vi "All-In-One_EIC-DIRC_DAQ.vi"() -> ()   [LabVIEW 2024]
uses:
  O:/DSG/Tyler/EIC/DIRC/daq/automated/Thorlabs.MotionControl.Controls.dll
  Thorlabs.MotionControl.Controls.dll
  <vilib>/numeric/Random Number (Range) DBL.vi
  O:/DSG/Tyler/EIC/DIRC/daq/automated/Thorlabs.MotionControl.IntegratedStepperMotorsCLI.dll
  Thorlabs.MotionControl.IntegratedStepperMotorsCLI.dll
  O:/DSG/Tyler/EIC/DIRC/daq/automated/Thorlabs.MotionControl.Benchtop.StepperMotorCLI.dll
  Thorlabs.MotionControl.Benchtop.StepperMotorCLI.dll
  <instrlib>/Keithley 6517/Keithley 6517.lvlib
panel:
  out "meter-mode":bool=TRUE
  in  "PDY start":dbl=105.8
  in  "PDX start":dbl=265.0
  out "run time (min)":dbl
  in  "align-only":bool
  out "alignment-counter":dbl=184.0 format="%#_13g"
  out "Optimized Location":dbl[](array[numeric])
  in  "N-M":bool
  in  "PD Y - in":cluster{"start":dbl, "stop":dbl, "step":dbl}={"start"=126.5, "stop"=128.5, "step"=2.0}
  in  "PD X - in":cluster{"start":dbl, "stop":dbl, "step":dbl}={"start"=268.0, "stop"=270.0, "step"=2.0}
  in  "out-pda":dbl=180.5 caption="Bar Out - PD Angle" format="%#_13g"
  in  "out-bma":dbl=45.0 caption="Bar Out - Brewster Angle" format="%#_13g"
  in  "out-bar-y":dbl=20.0 caption="Bar Out - Bar Y pos." format="%#_13g"
  in  "out-bar-x":dbl=93.0 caption="Bar Out - Bar X pos." format="%#_13g"
  in  "scan-v2":bool
  in  "in-pda":dbl=180.5 caption="Bar In - PD Angle" format="%#_13g"
  in  "in-bma":dbl=45.0 caption="Bar In - Brewster Angle" format="%#_13g"
  in  "Test Start Delay (s)":dbl=30.0
  in  "Bar Y - in":cluster{"start":dbl, "stop":dbl, "step":dbl}={"start"=20.0, "stop"=22.0, "step"=2.0}
  in  "Bar X - in":cluster{"start":dbl, "stop":dbl, "step":dbl}={"start"=235.0, "stop"=237.0, "step"=2.0}
  in  "PD Y - out":cluster{"start":dbl, "stop":dbl, "step":dbl}={"start"=126.5, "stop"=128.5, "step"=2.0}
  in  "PD X - out":cluster{"start":dbl, "stop":dbl, "step":dbl}={"start"=268.0, "stop"=270.0, "step"=2.0}
  out "Queue % Left":dbl format="%#_3g"
  out "next-state-cluster-const":T1={"next-state"="", "bypass-confirm"=FALSE, "PDX"=300.0, "PDY"=150.0, "BarX"=300.0, "BarY"=150.0, "BMA"=45.0, "PDA"=85.0, "bar-note"=FALSE}
  in  "X start":dbl=262.0
  in  "X end":dbl=263.0
  in  "Y end":dbl=121.5 format="%#_13g"
  in  "X step size":dbl=0.2 format="%#_13g"
  in  "Y step size":dbl=0.2
  in  "Y start":dbl=120.5 format="%#_13g"
  in  "diode-scan":bool
  out "keep-file":bool
  out "status":string
  out "queue-size":i32
  in  "save-loc":bool
  out "stored-pos":T2 caption="Location Stored"
  out "main-stage-refs":T3
  out "state-queue":T4(array[cluster])
  in  "PDA":dbl=184.0 format="%#_13g"
  in  "BMA":dbl=45.0 format="%#_13g"
  in  "BarY":dbl=30.0 format="%#_13g"
  in  "BarX":dbl=230.0 format="%#_13g"
  in  "PDY":dbl=124.0 format="%#_13g"
  in  "PDX":dbl=274.0 format="%#_13g"
  out "bypass-confirm":bool
  out "PD Values":cluster{"PD1":dbl, "PD2":dbl, "PD3":dbl}
  out "last-PD":dbl[](array[numeric])=[1.0, 1.0, 1.0]
  in  "move-bar":bool
  in  "multi-trial":bool
  out "pd_angle":dbl
  out "brewster_angle":dbl
  out "meter-visa":refnum<visa-resource-name>
  out "loop-rate":u32
  out "meter-stat":bool caption="Log Status"
  out "file-stat":bool caption="Log Status"
  out "stage-stat":bool caption="Log Status"
  out "last-save-time":string caption="Time of Last Save:"
  out "pd_y_pos":dbl
  out "pd_x_pos":dbl
  out "bar_y_pos":dbl
  out "bar_x_pos":dbl
  in  "nSamples":dbl=50.0 caption="# Samples"
  out "Current Time:":string
  in  "save-data":bool
  in  "bar-note":bool
  out "pd3_v":dbl caption="PD 3" format="%#.4g"
  out "pd2_v":dbl caption="PD 2" format="%#.4g"
  out "pd1_v":dbl caption="PD 1" format="%#.4g"
  out "meter-error":errorcluster
  out "log-error":errorcluster
  out "log-path":path caption="Path Data Will Save To:"
  out "start-msg":string
  out "stage-error":errorcluster
  in  "PD Angle":refnum<k24>(container)
  in  "Brewster":refnum<k24>(container)
  in  "PD Y":refnum<k24>(container)
  in  "PD X":refnum<k24>(container)
  in  "BAR Y":refnum<k24>(container)
  in  "stop":bool
  in  "BAR X":refnum<k24>(container)
  out "pd-plt":cluster{"[0]":dbl, "[1]":dbl, "[2]":dbl}(graph) caption="Measurement History"
  # "EXPERT DEBUGGING INFO"
  # "A"
  # "A"
  # "A"
  # "Work In Progress - please do not use"
  # "PD + BAR SCAN"
  # "BAR OUT SETTINGS"
  # "BAR IN SETTINGS"
  # "PD ONLY SCAN - CENTERED"
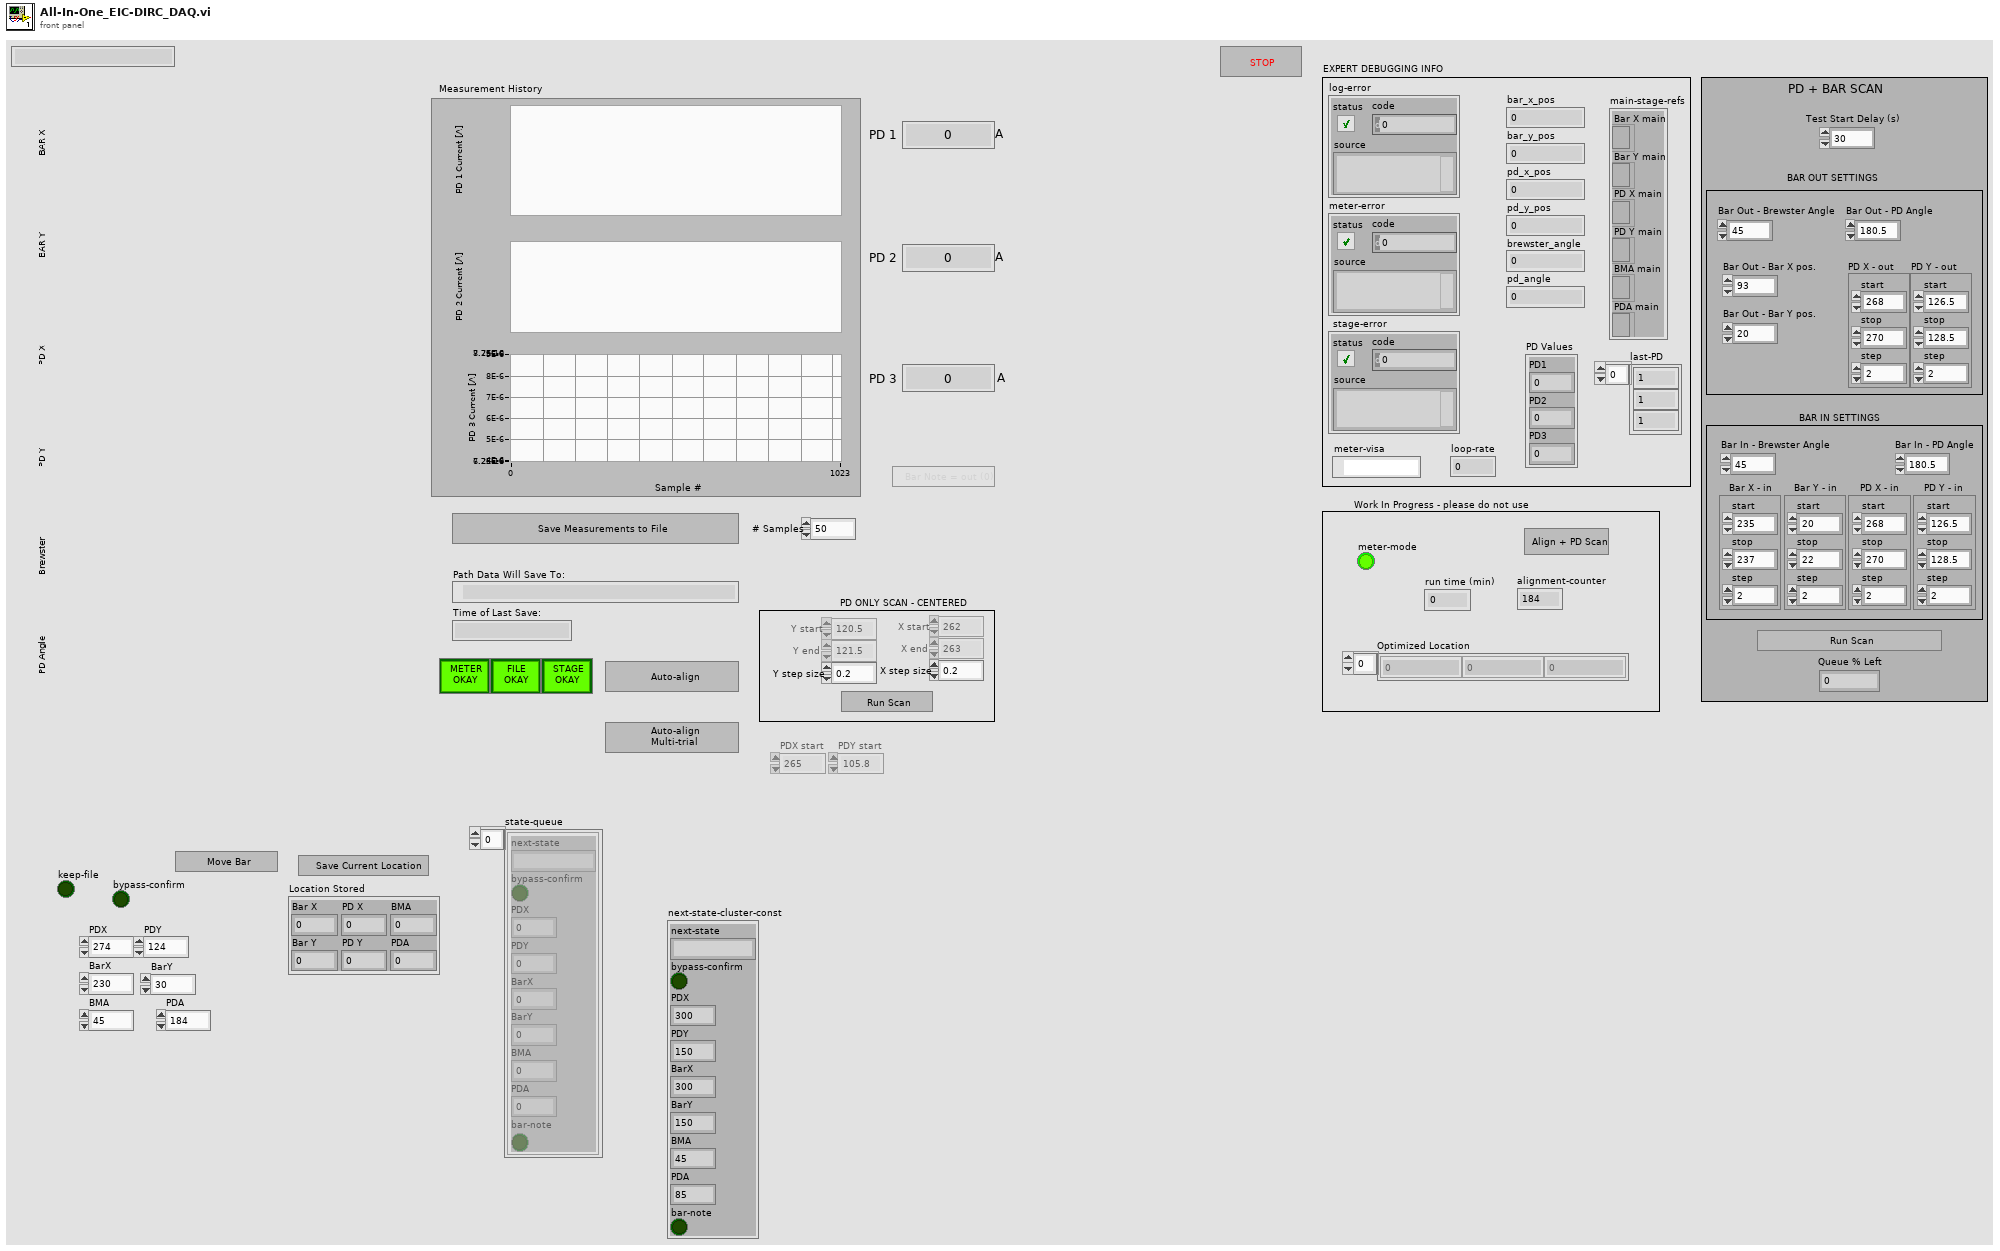
[diagram p1: front panel]
types:
  T1 = cluster{"next-state":string, "bypass-confirm":bool, "PDX":dbl, "PDY":dbl, "BarX":dbl, "BarY":dbl, "BMA":dbl, "PDA":dbl, "bar-note":bool}
  T2 = cluster{"Bar X":dbl, "Bar Y":dbl, "PD X":dbl, "PD Y":dbl, "BMA":dbl, "PDA":dbl}
  T3 = cluster{"Bar X main":refnum<k24>, "Bar Y main":refnum<k24>, "PD X main":refnum<k24>, "PD Y main":refnum<k24>, "BMA main":refnum<k24>, "PDA main":refnum<k24>}
  T4 = cluster{"next-state":string, "bypass-confirm":bool, "PDX":dbl, "PDY":dbl, "BarX":dbl, "BarY":dbl, "BMA":dbl, "PDA":dbl, "bar-note":bool}[]
  T5 = cluster{"Bar X":refnum<k24>, "Bar Y":refnum<k24>, "PD X":refnum<k24>, "PD Y":refnum<k24>, "Brewster":refnum<k24>, "PD Angle":refnum<k24>}
  T6 = enum16{"open", "replace", "create", "open or create", "replace or create", "replace or create with confirmation"}
  T7 = cluster{"alpha":dbl, "gamma":dbl, "rho":dbl, "sigma":dbl, "simplex L":dbl}
  T8 = cluster{"next-state":string, "mode-select":enum32{"IR", "Pure", "Bulk", "Bar Out", "stored-loc", "custom"}, "bypass-confirm":bool, "PDX":dbl, "PDY":dbl, "BarX":dbl, "BarY":dbl, "BMA":dbl, "PDA":dbl, "bar-note":bool}
  T9 = cluster{"error":bool, "code":i32, "source":string}
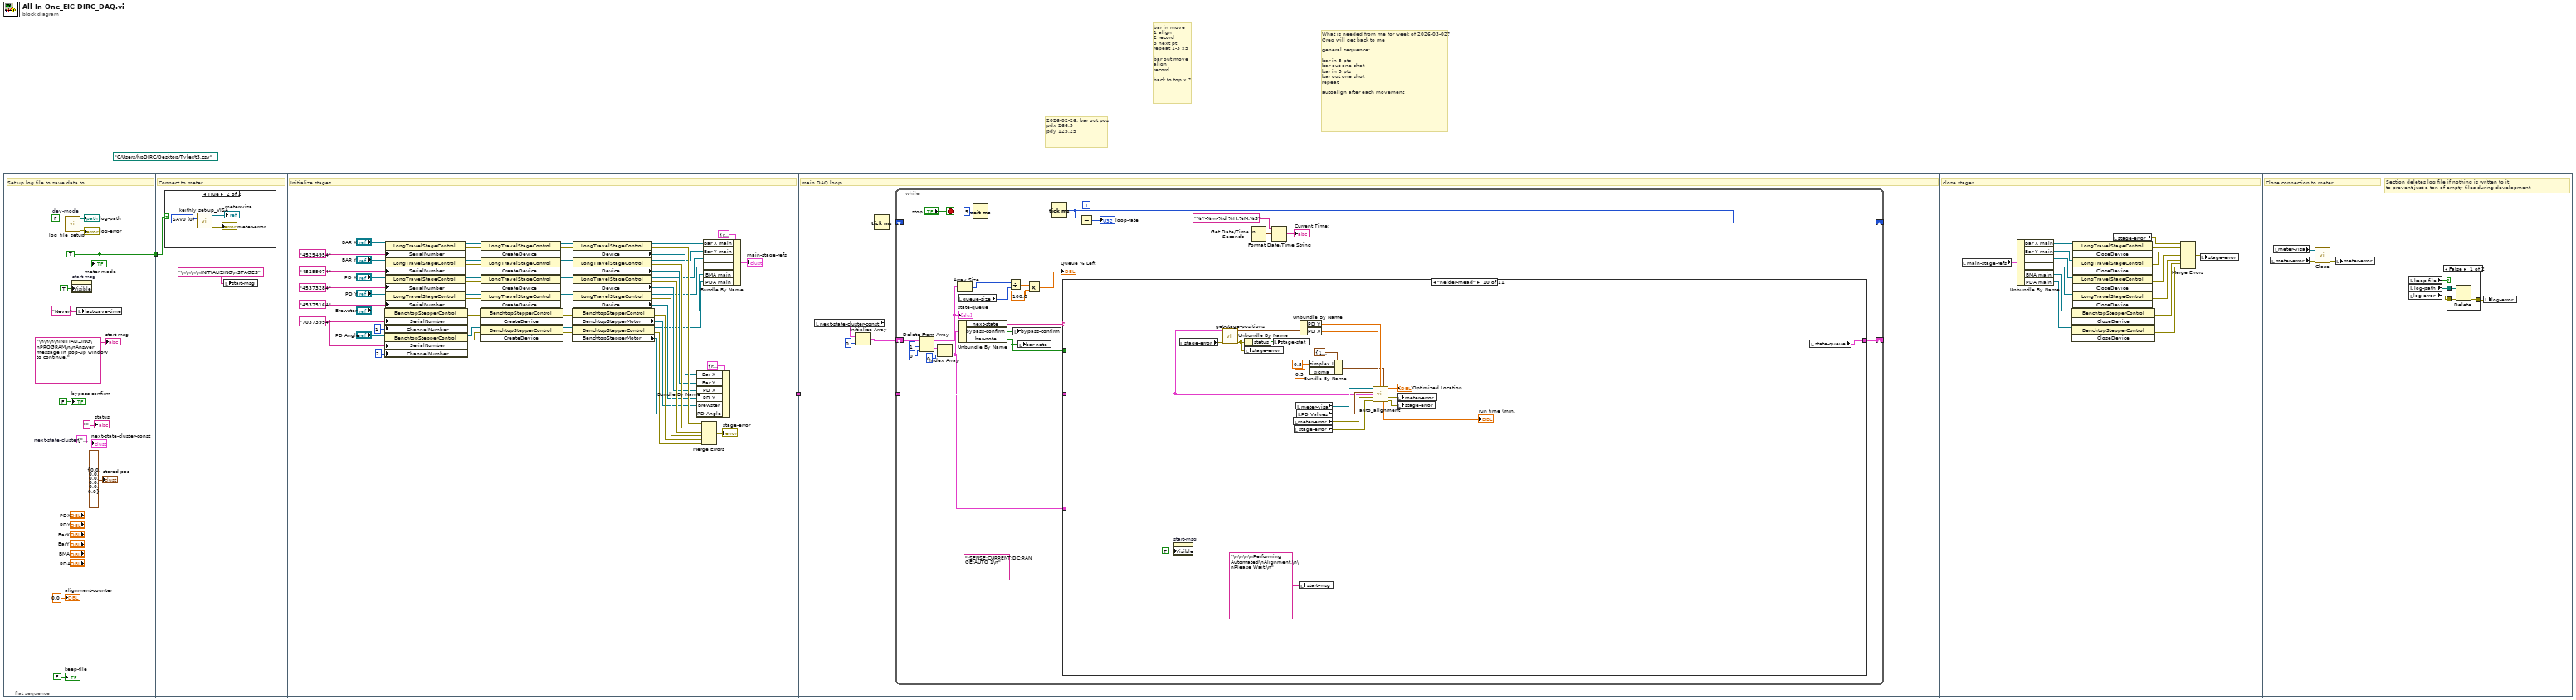
[diagram p0: block diagram]
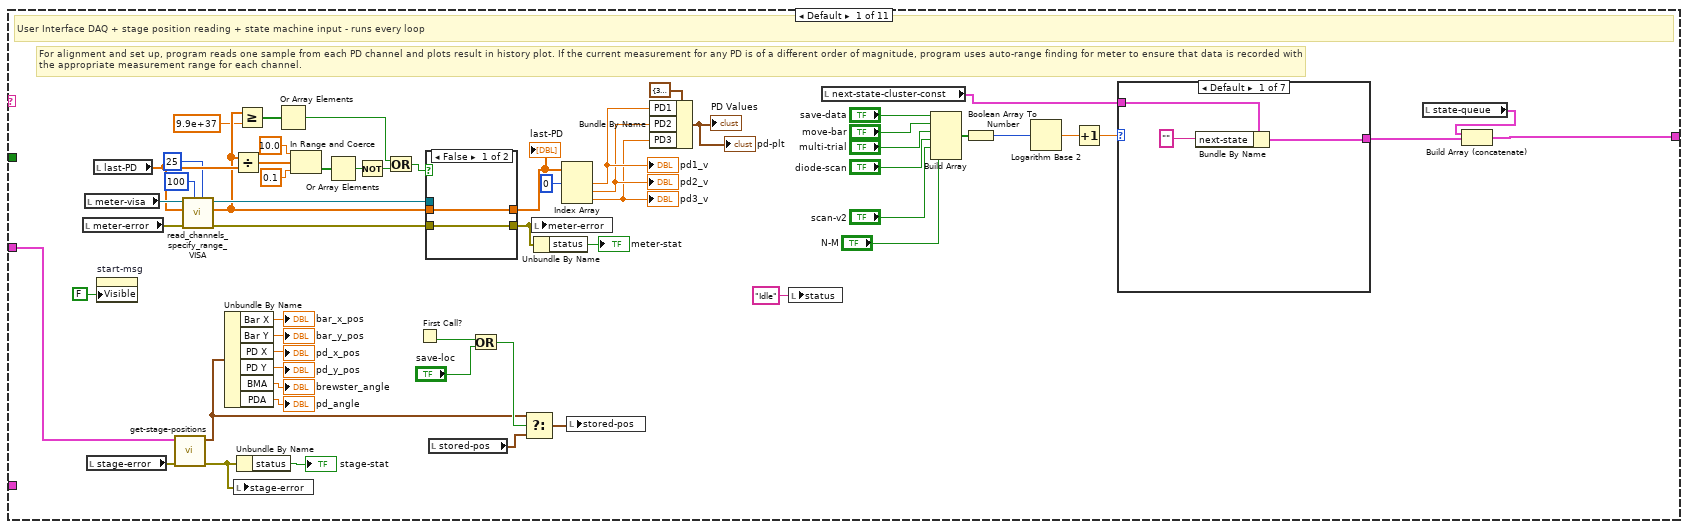
[diagram p3: hidden frame]
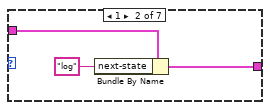
[diagram p4: hidden frame]
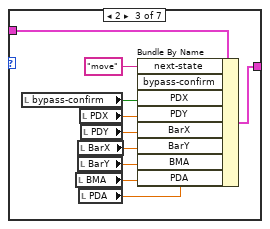
[diagram p5: hidden frame]
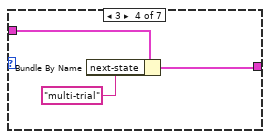
[diagram p6: hidden frame]
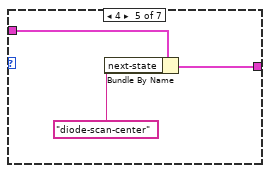
[diagram p7: hidden frame]
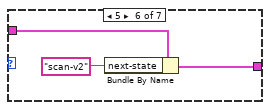
[diagram p8: hidden frame]
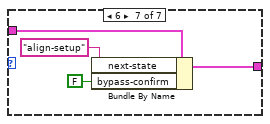
[diagram p9: hidden frame]
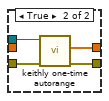
[diagram p10: hidden frame]
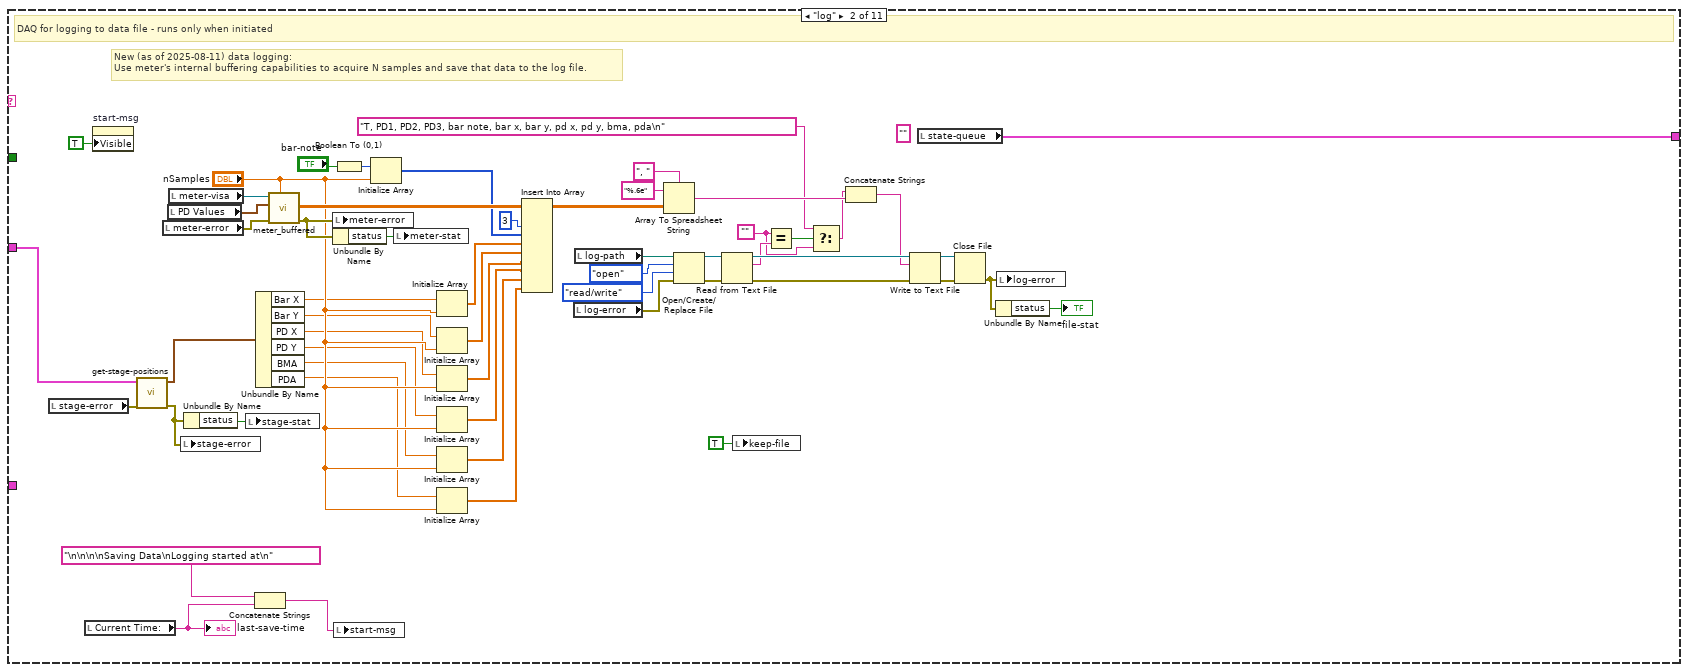
[diagram p11: hidden frame]
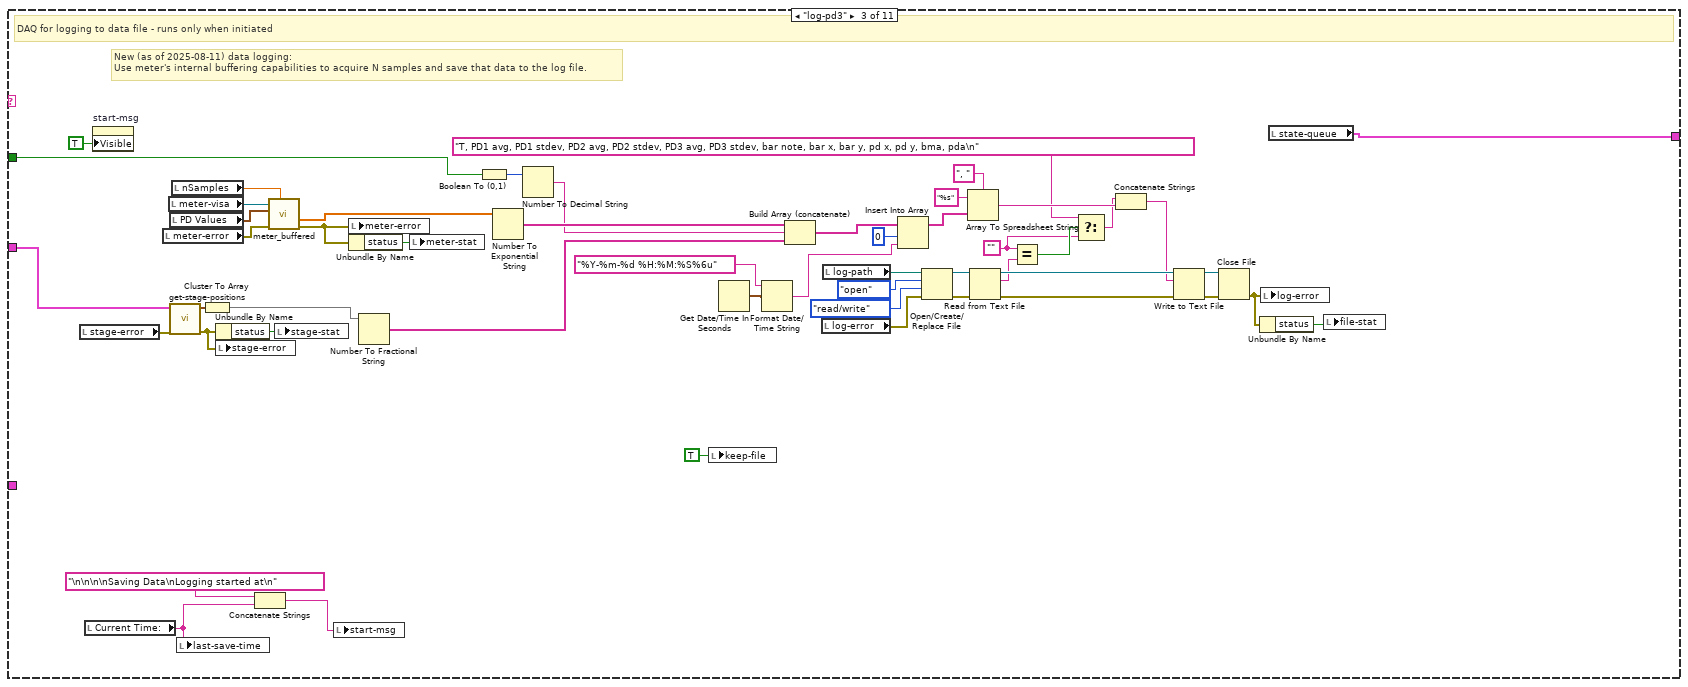
[diagram p12: hidden frame]
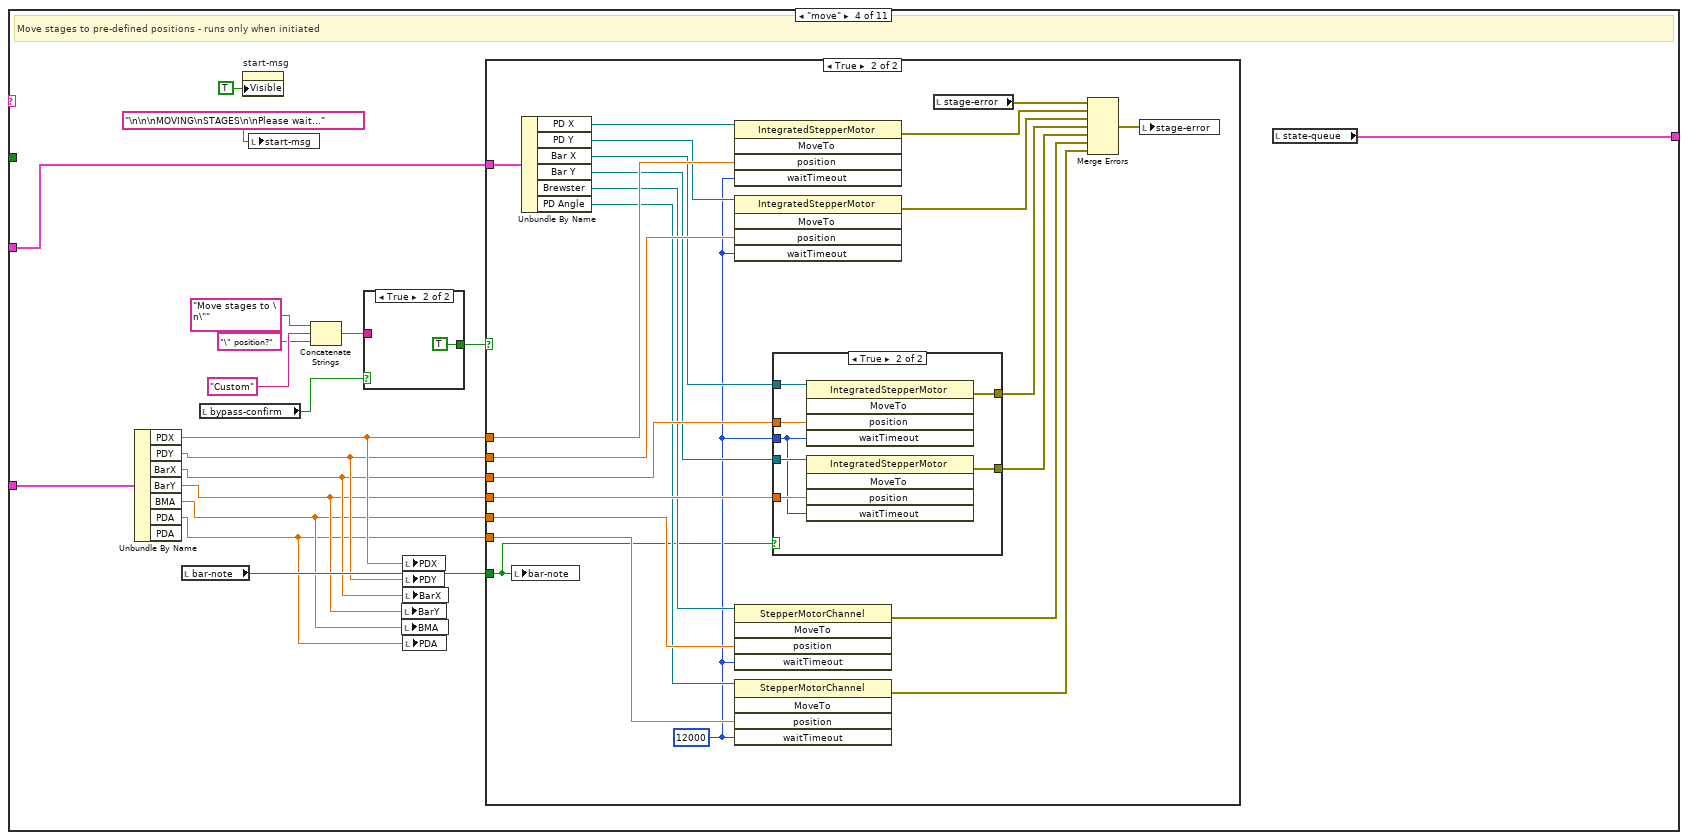
[diagram p13: hidden frame]
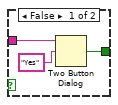
[diagram p14: hidden frame]
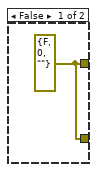
[diagram p16: hidden frame]
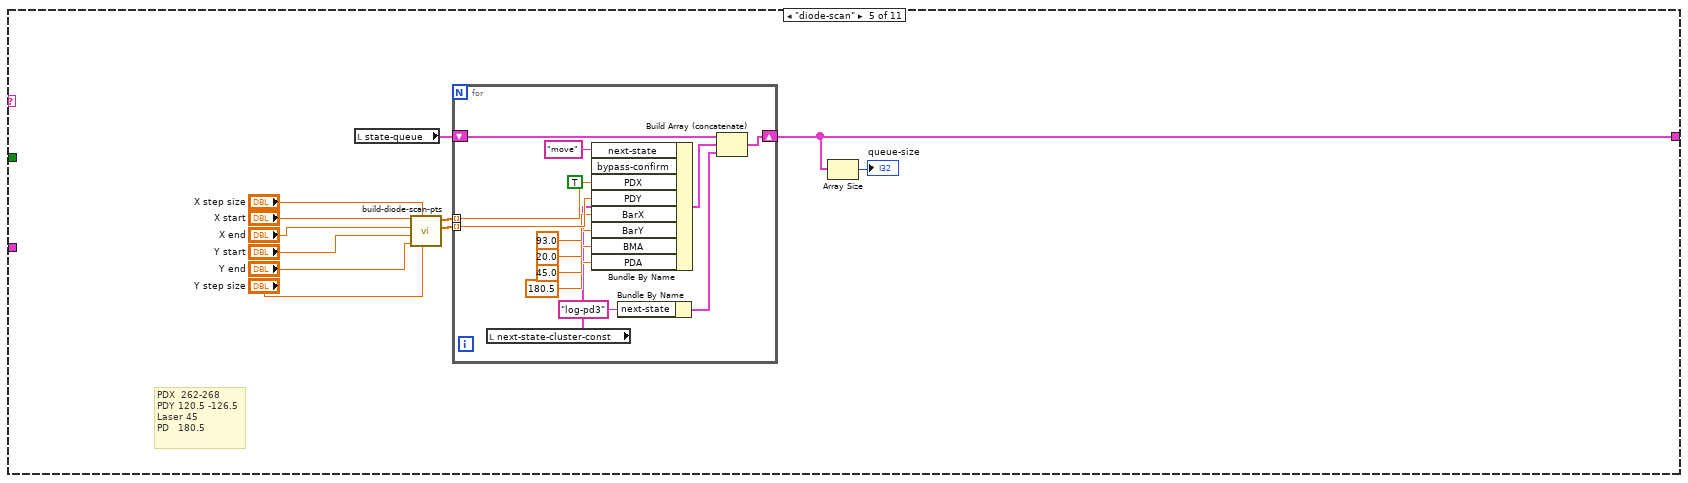
[diagram p17: hidden frame]
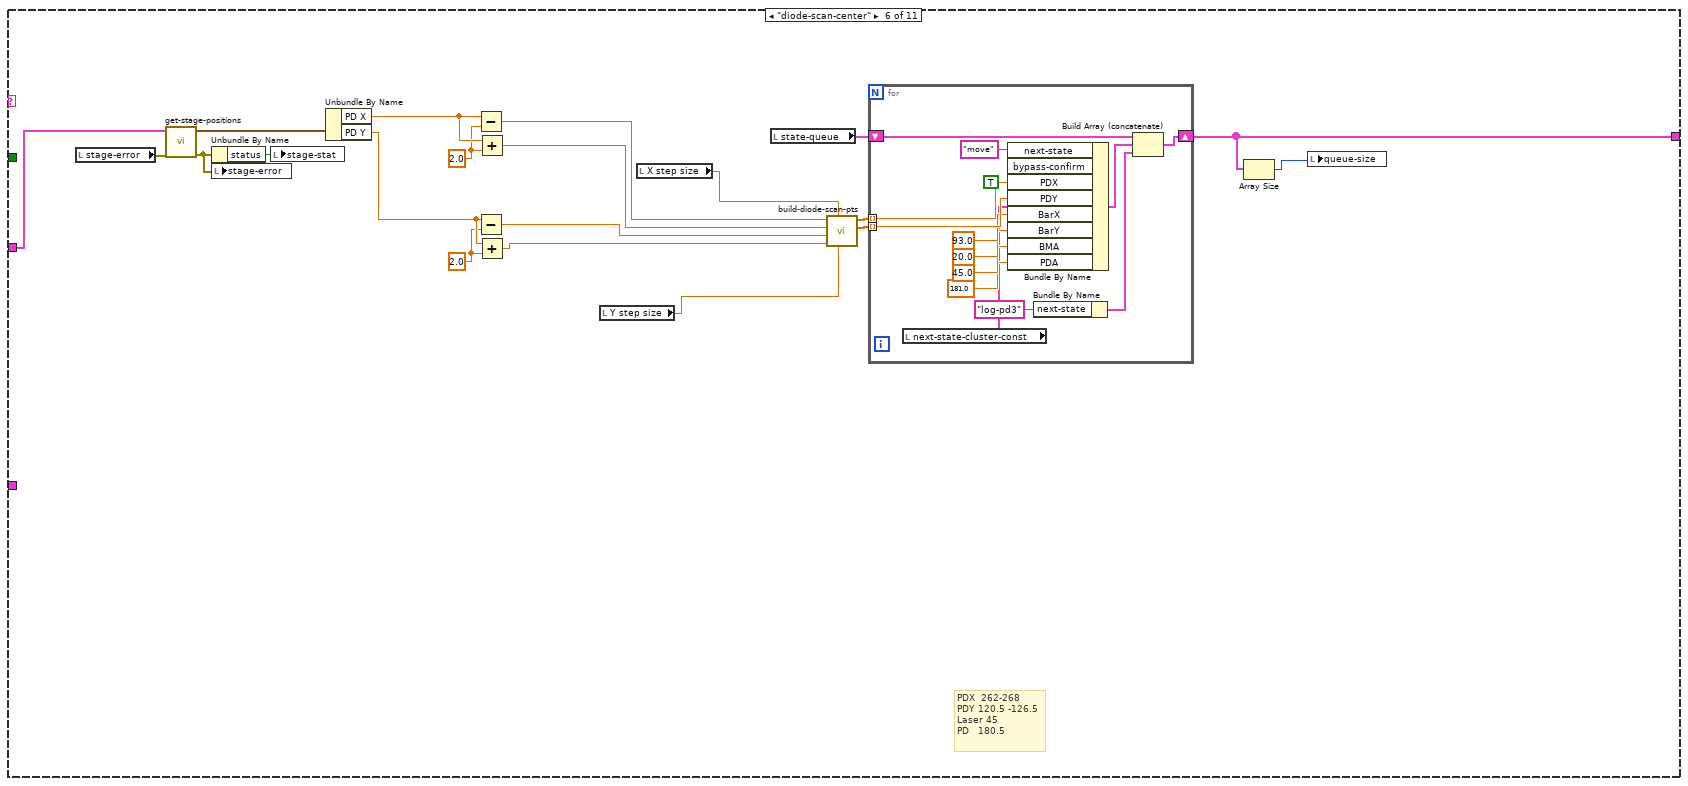
[diagram p18: hidden frame]
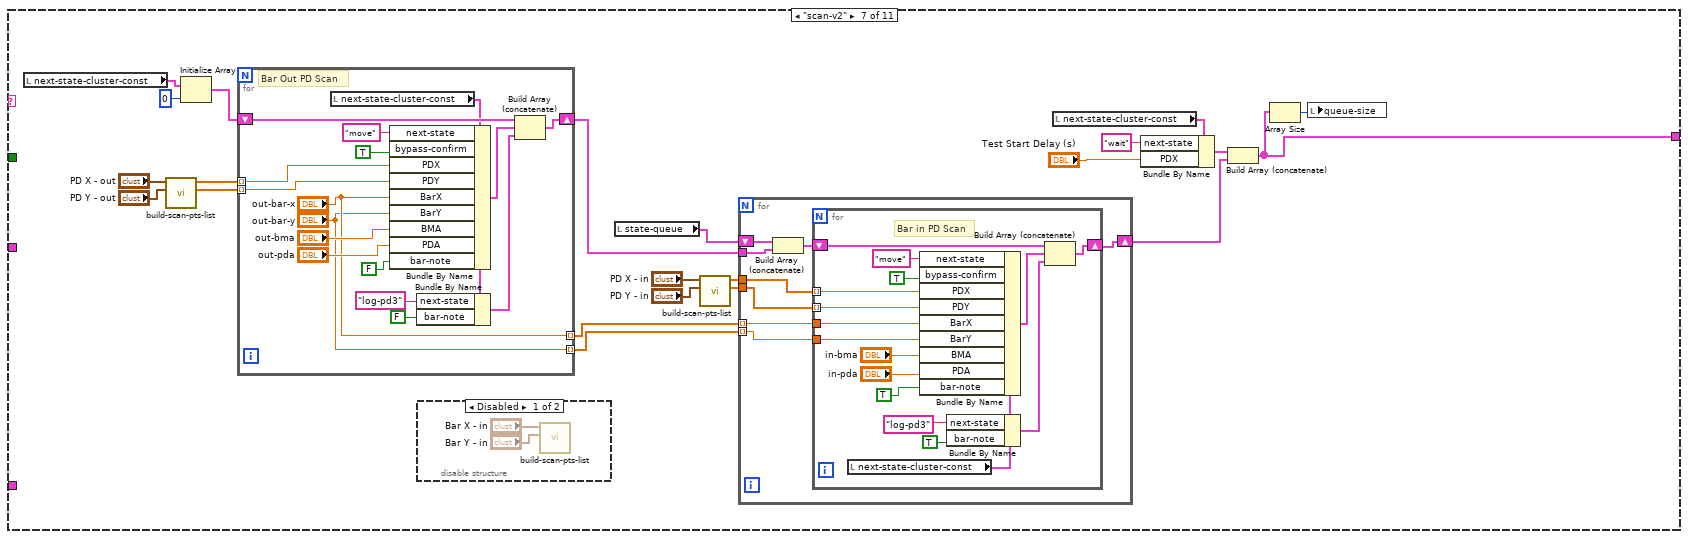
[diagram p19: hidden frame]
diagram:
  (unwired) path "C:/Users/hpDIRC/Desktop/Tyler/t3.csv" ("log-path")
  # "2026-02-26: bar out pos\npdx 266.5\npdy 125.25"
  # "bar in move\n1 align\n2 record\n3 next pt\nrepeat 1-3 x5\n\nbar out move\nalign\nrecord\n\nback to top x ?"
  # "What is needed from me for week of 2026-03-02?\nGreg will get back to me\n\ngeneral sequence:\n\nbar in 5 pts \nbar out one shot\nbar in 5 pts\nbar out one shot\nrepeat\n\nautoalign after each movement"
  n1 = flat-sequence {
    tunnel: [w3] -> w1
    tunnel: w1 -> [w15]
    tunnel: [w28] -> w2
    tunnel: w2 -> [w80]
    frame #0 {
      w3 = TRUE
      (unwired) T8 {"next-state"="", "mode-select"=enum."IR", "bypass-confirm"=FALSE, "PDX"=300.0, "PDY"=150.0, "BarX"=300.0, "BarY"=150.0, "BMA"=45.0, "PDA"=85.0, "bar-note"=FALSE}  # next-state-cluster
      w14 = FALSE  # dev-mode
      # "Set up log file to save data to"
      n2 = call "log_file_setup.vi"("dev-mode"=w14) -> ("error out"=→"log-error":errorcluster, "appended path"=→"log-path":path)  [unwired: 8 in, 1 out]
      n3 = property on="start-msg" class="Str"("Visible"=TRUE) -> ()  [unwired: 2 in, 2 out]
      n4 = local write "last-save-time"("Never" ("date/time string")) -> ()
      "start-msg" <- "\n\n\n\nINITIALIZING\nPROGRAM\n\nAnswer message in pop-up window to continue." ("String")
      "bypass-confirm" <- FALSE
      "stored-pos" <- T2 {"Bar X"=0.0, "Bar Y"=0.0, "PD X"=0.0, "PD Y"=0.0, "BMA"=0.0, "PDA"=0.0} ("stage-pos")
      "status" <- "" ("status")
      "keep-file" <- FALSE
      "alignment-counter" <- 0.0 ("alignment-counter")
      "meter-mode" <- w3
    }
    frame #1 {
      # "Connect to meter"
      n5 = case shown="True" w15 {
        frame False {
        }
        frame True {
          w17 = i16 0 items=["SAV0", "SAV1", "SAV2", "SAV3", "SAV4", "SAV5", "SAV6", "SAV7", "SAV8", "SAV9", "RST", "Preset"] ("ConfigOpt")
          n6 = call "keithly set-up_VISA.vi"("ConfigOpt"=w17) -> ("error out"=→"meter-error":errorcluster, "meter-VISA"=→"meter-visa":refnum<visa-resource-name>)  [unwired: 9 in]
        }
      }
      n7 = local write "start-msg"("\n\n\n\nINITIALIZING\nSTAGES" ("String")) -> ()
    }
    frame #2 {
      w35 = "70373994" ("SerialNumber")
      # "Initialize stages"
      n8 = property class="BenchtopStepperControl"(reference="Brewster", "SerialNumber"=w35, "ChannelNumber"=1) -> (reference out=w61:refnum<k24>, error out=w62:errorcluster)  [unwired: 1 in]
      n9 = property class="BenchtopStepperControl"(reference="PD Angle", "SerialNumber"=w35, "ChannelNumber"=2) -> (reference out=w60:refnum<k24>, error out=w63:errorcluster)  [unwired: 1 in]
      n10 = property class="LongTravelStageControl"(reference="BAR X", "SerialNumber"="45294954") -> (reference out=w38:refnum<k24>, error out=w45:errorcluster)  [unwired: 1 in]
      n11 = property class="LongTravelStageControl"(reference="BAR Y", "SerialNumber"="45299074") -> (reference out=w39:refnum<k24>, error out=w46:errorcluster)  [unwired: 1 in]
      n12 = property class="LongTravelStageControl"(reference="PD X", "SerialNumber"="45373284") -> (reference out=w42:refnum<k24>, error out=w47:errorcluster)  [unwired: 1 in]
      n13 = property class="LongTravelStageControl"(reference="PD Y", "SerialNumber"="45375164") -> (reference out=w43:refnum<k24>, error out=w48:errorcluster)  [unwired: 1 in]
      n14 = invoke class="BenchtopStepperControl" method="CreateDevice"(reference=w61, error in=w62) -> (reference out=w58:refnum<k24>, error out=w56:errorcluster)  [unwired: 1 in, 1 out]
      n15 = invoke class="BenchtopStepperControl" method="CreateDevice"(reference=w60, error in=w63) -> (reference out=w57:refnum<k24>, error out=w59:errorcluster)  [unwired: 1 in, 1 out]
      n16 = invoke class="LongTravelStageControl" method="CreateDevice"(reference=w38, error in=w45) -> (reference out=w51:refnum<k24>, error out=w55:errorcluster)  [unwired: 1 in, 1 out]
      n17 = invoke class="LongTravelStageControl" method="CreateDevice"(reference=w39, error in=w46) -> (reference out=w52:refnum<k24>)  [unwired: 1 in, 2 out]
      n18 = invoke class="LongTravelStageControl" method="CreateDevice"(reference=w42, error in=w47) -> (reference out=w53:refnum<k24>)  [unwired: 1 in, 2 out]
      n19 = invoke class="LongTravelStageControl" method="CreateDevice"(reference=w43, error in=w48) -> (reference out=w54:refnum<k24>)  [unwired: 1 in, 2 out]
      n20 = property class="BenchtopStepperControl"(reference=w58, error in=w56) -> (reference out=w22:refnum<k24>, error out=w73:errorcluster, "BenchtopStepperMotor"=w68:refnum<k24>)
      n21 = property class="BenchtopStepperControl"(reference=w57, error in=w59) -> (reference out=w21:refnum<k24>, error out=w74:errorcluster, "BenchtopStepperMotor"=w69:refnum<k24>)
      n22 = property class="LongTravelStageControl"(reference=w51, error in=w55) -> (reference out=w26:refnum<k24>, error out=w75:errorcluster, "Device"=w64:refnum<k24>)
      n23 = property class="LongTravelStageControl"(reference=w52) -> (reference out=w25:refnum<k24>, error out=w70:errorcluster, "Device"=w65:refnum<k24>)  [unwired: 1 in]
      n24 = property class="LongTravelStageControl"(reference=w53) -> (reference out=w24:refnum<k24>, error out=w71:errorcluster, "Device"=w66:refnum<k24>)  [unwired: 1 in]
      n25 = property class="LongTravelStageControl"(reference=w54) -> (reference out=w23:refnum<k24>, error out=w72:errorcluster, "Device"=w67:refnum<k24>)  [unwired: 1 in]
      n26 = Bundle By Name(cluster=T5 {"Bar X"=refnum, "Bar Y"=refnum, "PD X"=refnum, "PD Y"=refnum, "Brewster"=refnum, "PD Angle"=refnum}, "Bar X"=w64, "Bar Y"=w65, "PD X"=w66, "PD Y"=w67, "Brewster"=w68, "PD Angle"=w69) -> (w28:T5)
      n27 = Merge Errors(w75, w70, w71, w72, w73, w74) -> (→"stage-error":errorcluster)
      n28 = Bundle By Name(cluster=T3 {"Bar X main"=refnum, "Bar Y main"=refnum, "PD X main"=refnum, "PD Y main"=refnum, "BMA main"=refnum, "PDA main"=refnum}, "Bar X main"=w26, "Bar Y main"=w25, "PD X main"=w24, "PD Y main"=w23, "BMA main"=w22, "PDA main"=w21) -> (→"main-stage-refs":T3)
    }
    frame #3 {
      # "main DAQ loop"
      n29 = local read "next-state-cluster-const"() -> (w77:T1)
      n30 = Initialize Array(w77, 0 ("dimension size")) -> (w79:T4)
      n31 = Tick Count (ms)() -> (millisecond timer value=w81:u32)
      n32 = while {
        shift-right: [w105] -> _
        shift-left: w81 -> [w104]
        tunnel: w80 -> [w102]
        shift-right: [w90] -> _
        shift-left: w79 -> [w92]
        stop <- "stop" stop-if-true
        (unwired) ":SENSE:CURRENT:DC:RANGE:AUTO 1\n"
        n33 = Delete From Array(array=w92, length=1, index=0) -> (deleted portion=w91:T4, array with subset deleted=w88:T4)
        "state-queue" <- w88
        n34 = Index Array(array=w91, index=0) -> (element=w89:T1)
        n35 = Array Size(array=w88) -> (size(s)=w83:i32)
        n36 = local read "queue-size"() -> (w87:i32)
        n37 = Unbundle By Name(w89) -> ("next-state"=w94:string, "bypass-confirm"=w93:bool, "bar-note"=w82:bool)
        n38 = Wait (ms)(milliseconds to wait=u32 5) -> ()  [unwired: 1 out]
        n39 = Divide(x=w83, y=w87) -> (x/y=w86:dbl)
        n40 = local write "bypass-confirm"(w93) -> ()
        n41 = local write "bar-note"(w82) -> ()
        n42 = Multiply(x=w86, y=100.0) -> (x*y=→"Queue % Left":dbl)
        n43 = Tick Count (ms)() -> (millisecond timer value=w105:u32)
        n44 = case shown="\"nelder-mead\"" w94 {
          tunnel: w102 -> [w157 w218 w286 w319 _ w394 _ _ _ w526 _]
          tunnel: [w128 w229 w291 w317 w368 w402 w428 w486 w492 w534 w537] -> w90
          tunnel: w89 -> [_ _ _ w314 _ _ _ w487 w497 _ _]
          tunnel: w82 -> [_ _ w269 _ _ _ _ _ _ _ _]
          frame Default {
            # "For alignment and set up, program reads one sample from each PD channel and plots result in history plot. If the current measurement for any PD is of a different order of magnitude, program uses auto-range finding for meter to ensure that data is recorded with the appropriate measurement range for each channel."
            # "User Interface DAQ + stage position reading + state machine input - runs every loop"
            n45 = local read "meter-error"() -> (w154:errorcluster)
            n46 = local read "meter-visa"() -> (w155:refnum<visa-resource-name>)
            n47 = local read "stage-error"() -> (w156:errorcluster)
            n48 = local read "last-PD"() -> (w145:dbl[])
            n49 = property on="start-msg" class="Str"("Visible"=FALSE) -> ()  [unwired: 2 in, 2 out]
            n50 = call "get-stage-positions.vi"("error in (no error)"=w156, "Cluster"=w157) -> ("error out"=w142:errorcluster, "stage positions"=w114:T2)  [unwired: 8 in]
            n51 = call "read_channels_specify_range_VISA.vi"("postDAQ  wait ms"=u32 25, "preDAQ  wait ms"=u32 100, "error in"=w154, "range"=w145, "VISA resource in"=w155) -> ("error out"=w147:T9, "data"=w134:dbl[], "VISA resource out"=w146:refnum<visa-resource-name>)  [unwired: 4 in]
            n52 = Unbundle By Name(w114) -> ("Bar X"=→"bar_x_pos":dbl, "Bar Y"=→"bar_y_pos":dbl, "PD X"=→"pd_x_pos":dbl, "PD Y"=→"pd_y_pos":dbl, "BMA"=→"brewster_angle":dbl, "PDA"=→"pd_angle":dbl)
            n53 = Divide(x=w134, y=w145) -> (x/y=w150:dbl[])
            n54 = local write "stage-error"(w142) -> ()
            n55 = Greater Or Equal?(x=w134, y=9.9e+37) -> (x >= y?=w132:bool[])
            n56 = Unbundle By Name(w142) -> ("status"=→"stage-stat":bool)
            n57 = Or Array Elements(Boolean array=w132) -> (logical OR=w131:bool)
            n58 = In Range and Coerce(upper limit=10.0, x=w150, lower limit=0.1) -> (In Range?=w148:bool[])  [unwired: 1 out]
            n59 = Or Array Elements(Boolean array=w148) -> (logical OR=w149:bool)
            n60 = Not(x=w149) -> (.not. x?=w136:bool)
            n61 = Or(x=w131, y=w136) -> (x .or. y?=w135:bool)
            n62 = First Call?() -> (First Call?: T/F=w124:bool)
            n63 = case shown="False" w135 {
              tunnel: w147 -> [w196 w200]
              tunnel: [w196 w199] -> w163
              tunnel: [w195 w198] -> w158
              tunnel: w134 -> [w195 _]
              tunnel: w146 -> [_ w197]
              frame False {
              }
              frame True {
                n64 = call "keithly one-time autorange.vi"("error in"=w200, "VISA in"=w197) -> ("error out"=w199:errorcluster, "data"=w198:dbl[])  [unwired: 7 in, 1 out]
              }
            }
            "last-PD" <- w158
            n65 = local read "stored-pos"() -> (w125:T2)
            n66 = Or(x=w124, y="save-loc") -> (x .or. y?=w122:bool)
            n67 = Select(t=w114, s=w122, f=w125) -> (s? t:f=w126:T2)
            n68 = local write "meter-error"(w163) -> ()
            n69 = Unbundle By Name(w163) -> ("status"=→"meter-stat":bool)
            n70 = Index Array(array=w158, index #1=0 ("index")) -> (element #1=w161:dbl, element #2=w160:dbl, element #3=w159:dbl)  [unwired: 2 in]
            "pd3_v" <- w159
            "pd2_v" <- w160
            "pd1_v" <- w161
            n71 = local write "stored-pos"(w126) -> ()
            n72 = Bundle By Name(cluster=cluster{"PD1":dbl, "PD2":dbl, "PD3":dbl} {"PD1"=3e-05, "PD2"=3e-05, "PD3"=3e-05} ("PD ranges"), "PD1"=w161, "PD2"=w160, "PD3"=w159) -> (→"pd-plt" →"PD Values":cluster{"PD1":dbl, "PD2":dbl, "PD3":dbl})
            n73 = local write "status"("Idle" ("status")) -> ()
            n74 = local read "next-state-cluster-const"() -> (w112:T1)
            n75 = Build Array("save-data", "move-bar", "multi-trial", "diode-scan", "scan-v2", "N-M") -> (w138:bool[])
            n76 = Boolean Array To Number(Boolean array=w138) -> (number=w108:u32)
            n77 = Logarithm Base 2(1:w108) -> (0:w110:dbl)
            n78 = Increment(x=w110) -> (x+1=w109:dbl)
            n79 = case shown="Default" w109 {
              tunnel: w112 -> [w168 w171 w181 w184 w187 w190 w193]
              tunnel: [w166 w169 w179 w182 w185 w188 w194] -> w127
              frame Default {
                n80 = Bundle By Name(cluster=w168, "next-state"="") -> (w166:T1)
              }
              frame 1 {
                n81 = Bundle By Name(cluster=w171, "next-state"="log") -> (w169:T1)
              }
              frame 2 {
                n82 = local read "bypass-confirm"() -> (w172:bool)
                n83 = local read "BMA"() -> (w177:dbl)
                n84 = local read "BarX"() -> (w175:dbl)
                n85 = local read "BarY"() -> (w176:dbl)
                n86 = local read "PDA"() -> (w178:dbl)
                n87 = local read "PDX"() -> (w173:dbl)
                n88 = local read "PDY"() -> (w174:dbl)
                n89 = Bundle By Name(cluster=w181, "next-state"="move", "bypass-confirm"=w172, "PDX"=w173, "PDY"=w174, "BarX"=w175, "BarY"=w176, "BMA"=w177, "PDA"=w178) -> (w179:T1)
              }
              frame 3 {
                n90 = Bundle By Name(cluster=w184, "next-state"="multi-trial") -> (w182:T1)
              }
              frame 4 {
                n91 = Bundle By Name(cluster=w187, "next-state"="diode-scan-center") -> (w185:T1)
              }
              frame 5 {
                n92 = Bundle By Name(cluster=w190, "next-state"="scan-v2") -> (w188:T1)
              }
              frame 6 {
                n93 = Bundle By Name(cluster=w193, "next-state"="align-setup", "bypass-confirm"=FALSE) -> (w194:T1)
              }
            }
            n94 = local read "state-queue"() -> (w129:T4)
            n95 = Build Array (concatenate)(w129, w127) -> (w128:T4)
          }
          frame "log" {
            w204 = ""
            (unwired) ""
            # "New (as of 2025-08-11) data logging:\nUse meter's internal buffering capabilities to acquire N samples and save that data to the log file."
            # "DAQ for logging to data file - runs only when initiated"
            n96 = local read "stage-error"() -> (w217:errorcluster)
            n97 = local read "Current Time:"() -> (w227:string)
            "last-save-time" <- w227
            n98 = property on="start-msg" class="Str"("Visible"=TRUE) -> ()  [unwired: 2 in, 2 out]
            n99 = call "get-stage-positions.vi"("error in (no error)"=w217, "Cluster"=w218) -> ("error out"=w216:errorcluster, "stage positions"=w214:T2)  [unwired: 8 in]
            n100 = local read "meter-error"() -> (w255:errorcluster)
            n101 = local read "PD Values"() -> (w232:cluster{"PD1":dbl, "PD2":dbl, "PD3":dbl})
            n102 = local read "meter-visa"() -> (w256:refnum<visa-resource-name>)
            n103 = local write "stage-error"(w216) -> ()
            n104 = Unbundle By Name(w216) -> ("status"=w215:bool)
            n105 = local write "stage-stat"(w215) -> ()
            n106 = Concatenate Strings("\n\n\n\nSaving Data\nLogging started at\n" ("String"), w227) -> (w230:string)
            n107 = Unbundle By Name(w214) -> ("Bar X"=w213:dbl, "Bar Y"=w212:dbl, "PD X"=w211:dbl, "PD Y"=w210:dbl, "BMA"=w209:dbl, "PDA"=w208:dbl)
            n108 = call "meter_buffered.vi"("Samples"="nSamples", "error in"=w255, "PD ranges"=w232, "meter-VISA"=w256) -> ("error out"=w233:errorcluster, "ch1-3 data"=w243:dbl[][])  [unwired: 3 in, 3 out]
            n109 = local write "meter-error"(w233) -> ()
            n110 = Unbundle By Name(w233) -> ("status"=w234:bool)
            n111 = Boolean To (0,1)(Boolean="bar-note") -> (0, 1=w240:i16)
            n112 = local write "start-msg"(w230) -> ()
            n113 = Initialize Array(w240, "nSamples") -> (w241:i16[])
            n114 = local write "meter-stat"(w234) -> ()
            n115 = Initialize Array(w213, "nSamples") -> (w224:dbl[])
            n116 = Initialize Array(w212, "nSamples") -> (w223:dbl[])
            n117 = Initialize Array(w211, "nSamples") -> (w222:dbl[])
            n118 = Initialize Array(w210, "nSamples") -> (w221:dbl[])
            n119 = Initialize Array(w209, "nSamples") -> (w220:dbl[])
            n120 = Initialize Array(w208, "nSamples") -> (w219:dbl[])
            n121 = Insert Into Array(array=w243, index (col)=3 ("disabled index (col)"), new element #1=w241, new element #2=w224, new element #3=w223, new element #4=w222, new element #5=w221, new element #6=w220, new element #7=w219) -> (w226:dbl[][])  [unwired: 1 in]
            n122 = local read "log-error"() -> (w253:errorcluster)
            n123 = local read "log-path"() -> (w254:path)
            n124 = Array To Spreadsheet String(delimiter (Tab)=", ", array=w226, 3:"%.6e" ("format string")) -> (spreadsheet string=w237:string)
            n125 = Open/Create/Replace File(file path (use dialog)=w254, error in=w253, operation (0:open)=T6."open", access (0:read/write)=enum16{"read/write", "read-only", "write-only"}."read/write") -> (refnum out=w252:refnum<file>, error out=w248:errorcluster)  [unwired: 2 in, 1 out]
            n126 = Read from Text File(file (use dialog)=w252, error in=w248) -> (refnum out=w249:refnum<file>, text=w206:string, error out=w247:errorcluster)  [unwired: 2 in, 1 out]
            n127 = local write "keep-file"(TRUE ("keep-file")) -> ()
            n128 = Equal?(x=w204, y=w206) -> (x = y?=w205:bool)
            n129 = Select(t="T, PD1, PD2, PD3, bar note, bar x, bar y, pd x, pd y, bma, pda\n", s=w205, f=w204) -> (s? t:f=w201:string)
            n130 = Concatenate Strings(w201, w237) -> (w202:string)
            n131 = Write to Text File(file (use dialog)=w249, text=w202, error in=w247) -> (refnum out=w251:refnum<file>, error out=w250:errorcluster)  [unwired: 1 in, 1 out]
            n132 = local read "state-queue"() -> (w229:T4)
            n133 = Close File(refnum=w251, error in=w250) -> (error out=w246:errorcluster)  [unwired: 1 out]
            n134 = Unbundle By Name(w246) -> ("status"=→"file-stat":bool)
            n135 = local write "log-error"(w246) -> ()
          }
          frame "log-pd3" {
            w271 = ""
            # "New (as of 2025-08-11) data logging:\nUse meter's internal buffering capabilities to acquire N samples and save that data to the log file."
            # "DAQ for logging to data file - runs only when initiated"
            n136 = local read "stage-error"() -> (w285:errorcluster)
            n137 = local read "Current Time:"() -> (w289:string)
            n138 = property on="start-msg" class="Str"("Visible"=TRUE) -> ()  [unwired: 2 in, 2 out]
            n139 = local read "meter-error"() -> (w258:errorcluster)
            n140 = local read "meter-visa"() -> (w260:refnum<visa-resource-name>)
            n141 = local read "PD Values"() -> (w259:cluster{"PD1":dbl, "PD2":dbl, "PD3":dbl})
            n142 = call "get-stage-positions.vi"("error in (no error)"=w285, "Cluster"=w286) -> ("error out"=w284:errorcluster, "stage positions"=w283:T2)  [unwired: 8 in]
            n143 = local read "nSamples"() -> (w261:dbl)
            n144 = local write "last-save-time"(w289) -> ()
            n145 = Cluster To Array(cluster=w283) -> (array=w268:dbl[])
            n146 = Unbundle By Name(w284) -> ("status"=w287:bool)
            n147 = local write "stage-error"(w284) -> ()
            n148 = Concatenate Strings("\n\n\n\nSaving Data\nLogging started at\n" ("String"), w289) -> (w292:string)
            n149 = call "meter_buffered.vi"("Samples"=w261, "error in"=w258, "PD ranges"=w259, "meter-VISA"=w260) -> ("error out"=w262:errorcluster, "stats-out"=w257:dbl[])  [unwired: 3 in, 3 out]
            n150 = local write "stage-stat"(w287) -> ()
            n151 = local write "start-msg"(w292) -> ()
            n152 = local write "meter-error"(w262) -> ()
            n153 = Unbundle By Name(w262) -> ("status"=w294:bool)
            n154 = Number To Fractional String(number=w268) -> (F-format string=w263:string[])  [unwired: 3 in]
            n155 = local write "meter-stat"(w294) -> ()
            n156 = Boolean To (0,1)(Boolean=w269) -> (0, 1=w267:i16)
            n157 = Number To Exponential String(number=w257) -> (E-format string=w266:string[])  [unwired: 3 in]
            n158 = Number To Decimal String(number=w267) -> (decimal integer string=w264:string)  [unwired: 1 in]
            n159 = local write "keep-file"(TRUE ("keep-file")) -> ()
            n160 = Get Date/Time In Seconds() -> (seconds since 1Jan1904=w282:timestamp)
            n161 = Format Date/Time String(time format string (%c)="%Y-%m-%d %H:%M:%S%6u", seconds (now)=w282) -> (date/time string=w278:string)  [unwired: 1 in]
            n162 = Build Array (concatenate)(w266, w264, w263) -> (w265:string[])
            n163 = local read "log-error"() -> (w306:errorcluster)
            n164 = local read "log-path"() -> (w307:path)
            n165 = Insert Into Array(array=w265, index=0, new element=w278) -> (w279:string[])
            n166 = Open/Create/Replace File(file path (use dialog)=w307, error in=w306, operation (0:open)=T6."open", access (0:read/write)=enum16{"read/write", "read-only", "write-only"}."read/write") -> (refnum out=w305:refnum<file>, error out=w301:errorcluster)  [unwired: 2 in, 1 out]
            n167 = Array To Spreadsheet String(delimiter (Tab)=", ", array=w279, 3:"%s" ("format string")) -> (spreadsheet string=w295:string)
            n168 = Read from Text File(file (use dialog)=w305, error in=w301) -> (refnum out=w302:refnum<file>, text=w275:string, error out=w300:errorcluster)  [unwired: 2 in, 1 out]
            n169 = Equal?(x=w271, y=w275) -> (x = y?=w272:bool)
            n170 = Select(t="T, PD1 avg, PD1 stdev, PD2 avg, PD2 stdev, PD3 avg, PD3 stdev, bar note, bar x, bar y, pd x, pd y, bma, pda\n", s=w272, f=w271) -> (s? t:f=w273:string)
            n171 = Concatenate Strings(w273, w295) -> (w274:string)
            n172 = Write to Text File(file (use dialog)=w302, text=w274, error in=w300) -> (refnum out=w304:refnum<file>, error out=w303:errorcluster)  [unwired: 1 in, 1 out]
            n173 = Close File(refnum=w304, error in=w303) -> (error out=w299:errorcluster)  [unwired: 1 out]
            n174 = Unbundle By Name(w299) -> ("status"=w288:bool)
            n175 = local write "log-error"(w299) -> ()
            n176 = local read "state-queue"() -> (w291:T4)
            n177 = local write "file-stat"(w288) -> ()
          }
          frame "move" {
            # "Move stages to pre-defined positions - runs only when initiated"
            n178 = Unbundle By Name(w314) -> ("PDX"=w313:dbl, "PDY"=w312:dbl, "BarX"=w311:dbl, "BarY"=w310:dbl, "BMA"=w309:dbl, "PDA"=w308:dbl)  [unwired: 1 out]
            n179 = local read "bar-note"() -> (w325:bool)
            n180 = local read "bypass-confirm"() -> (w318:bool)
            n181 = property on="start-msg" class="Str"("Visible"=TRUE) -> ()  [unwired: 2 in, 2 out]
            n182 = local write "start-msg"("\n\n\nMOVING\nSTAGES\n\nPlease wait..." ("String")) -> ()
            n183 = Concatenate Strings("Move stages to \n\"", "Custom", "\" position?" ("string")) -> (w321:string)
            n184 = case shown="True" w318 {
              tunnel: [w328 TRUE ("T button?")] -> w324
              tunnel: w321 -> [w327 _]
              frame False {
                n185 = Two Button Dialog(message=w327, 2:"Yes" ("T button name (\"OK\")")) -> (T button?=w328:bool)  [unwired: 1 in]
              }
              frame True {
              }
            }
            n186 = local write "BarY"(w310) -> ()
            n187 = local write "BMA"(w309) -> ()
            n188 = local write "PDX"(w313) -> ()
            n189 = local write "PDY"(w312) -> ()
            n190 = local write "BarX"(w311) -> ()
            n191 = local write "PDA"(w308) -> ()
            n192 = case shown="True" w324 {
              tunnel: w313 -> [_ w344]
              tunnel: w312 -> [_ w343]
              tunnel: w311 -> [_ w342]
              tunnel: w310 -> [_ w341]
              tunnel: w309 -> [_ w340]
              tunnel: w308 -> [_ w339]
              tunnel: w325 -> [_ w330]
              tunnel: w319 -> [_ w338]
              frame False {
              }
              frame True {
                w331 = 12000 ("waitTimeout")
                n193 = local write "bar-note"(w330) -> ()
                n194 = Unbundle By Name(w338) -> ("PD X"=w337:refnum<k24>, "PD Y"=w332:refnum<k24>, "Bar X"=w333:refnum<k24>, "Bar Y"=w334:refnum<k24>, "Brewster"=w335:refnum<k24>, "PD Angle"=w336:refnum<k24>)
                n195 = invoke class="IntegratedStepperMotor" method="MoveTo"(reference=w337, "position"=w344, "waitTimeout"=w331) -> (error out=w351:errorcluster)  [unwired: 2 in, 4 out]
                n196 = invoke class="IntegratedStepperMotor" method="MoveTo"(reference=w332, "position"=w343, "waitTimeout"=w331) -> (error out=w350:errorcluster)  [unwired: 2 in, 4 out]
                n197 = invoke class="StepperMotorChannel" method="MoveTo"(reference=w335, "position"=w340, "waitTimeout"=w331) -> (error out=w347:errorcluster)  [unwired: 2 in, 4 out]
                n198 = invoke class="StepperMotorChannel" method="MoveTo"(reference=w336, "position"=w339, "waitTimeout"=w331) -> (error out=w346:errorcluster)  [unwired: 2 in, 4 out]
                n199 = case shown="True" w330 {
                  tunnel: [w353 w360] -> w349
                  tunnel: [w353 w359] -> w348
                  tunnel: w342 -> [_ w358]
                  tunnel: w341 -> [_ w357]
                  tunnel: w334 -> [_ w356]
                  tunnel: w333 -> [_ w355]
                  tunnel: w331 -> [_ w354]
                  frame False {
                    w353 = errorcluster {"status"=FALSE, "code"=0, "source"=""} ("error out")
                  }
                  frame True {
                    n200 = invoke class="IntegratedStepperMotor" method="MoveTo"(reference=w355, "position"=w358, "waitTimeout"=w354) -> (error out=w360:errorcluster)  [unwired: 2 in, 4 out]
                    n201 = invoke class="IntegratedStepperMotor" method="MoveTo"(reference=w356, "position"=w357, "waitTimeout"=w354) -> (error out=w359:errorcluster)  [unwired: 2 in, 4 out]
                  }
                }
                n202 = local read "stage-error"() -> (w352:errorcluster)
                n203 = Merge Errors(w352, w351, w350, w349, w348, w347, w346) -> (w345:errorcluster)
                n204 = local write "stage-error"(w345) -> ()
              }
            }
            n205 = local read "state-queue"() -> (w317:T4)
          }
          frame "diode-scan" {
            # "PDX  262-268\nPDY 120.5 -126.5\nLaser 45\nPD   180.5"
            n206 = local read "state-queue"() -> (w371:T4)
            n207 = call "build-diode-scan-pts.vi"("Y step size"="Y step size", "X step size"="X step size", "Y end"="Y end", "Y start"="Y start", "X end"="X end", "X start"="X start") -> ("y"=w369:dbl[], "x"=w370:dbl[])  [unwired: 4 in]
            n208 = for {
              tunnel: w370 -> [w385] mode=indexing
              tunnel: w369 -> [w384] mode=indexing
              shift-right: [w378] -> w368
              shift-left: w371 -> [w380]
              n209 = local read "next-state-cluster-const"() -> (w372:T1)
              n210 = Bundle By Name(cluster=w372, "next-state"="move", "bypass-confirm"=TRUE, "PDX"=w385, "PDY"=w384, "BarX"=93.0, "BarY"=20.0, "BMA"=45.0, "PDA"=180.5) -> (w379:T1)
              n211 = Bundle By Name(cluster=w372, "next-state"="log-pd3") -> (w373:T1)
              n212 = Build Array (concatenate)(w380, w379, w373) -> (w378:T4)
            }
            n213 = Array Size(array=w368) -> (size(s)=→"queue-size":i32)
          }
          frame "diode-scan-center" {
            w389 = 2.0 ("y")
            w388 = 2.0 ("y")
            # "PDX  262-268\nPDY 120.5 -126.5\nLaser 45\nPD   180.5"
            n214 = local read "stage-error"() -> (w397:errorcluster)
            n215 = call "get-stage-positions.vi"("error in (no error)"=w397, "Cluster"=w394) -> ("error out"=w396:errorcluster, "stage positions"=w395:T2)  [unwired: 8 in]
            n216 = Unbundle By Name(w396) -> ("status"=w398:bool)
            n217 = local write "stage-error"(w396) -> ()
            n218 = local write "stage-stat"(w398) -> ()
            n219 = Unbundle By Name(w395) -> ("PD X"=w393:dbl, "PD Y"=w390:dbl)
            n220 = Subtract(x=w393, y=w388) -> (x-y=w392:dbl)
            n221 = Subtract(x=w390, y=w389) -> (x-y=w387:dbl)
            n222 = Add(x=w393, y=w388) -> (x+y=w391:dbl)
            n223 = Add(x=w390, y=w389) -> (x+y=w386:dbl)
            n224 = local read "Y step size"() -> (w400:dbl)
            n225 = local read "X step size"() -> (w401:dbl)
            n226 = local read "state-queue"() -> (w405:T4)
            n227 = call "build-diode-scan-pts.vi"("Y step size"=w400, "X step size"=w401, "Y end"=w386, "Y start"=w387, "X end"=w391, "X start"=w392) -> ("y"=w403:dbl[], "x"=w404:dbl[])  [unwired: 4 in]
            n228 = for {
              tunnel: w404 -> [w419] mode=indexing
              tunnel: w403 -> [w418] mode=indexing
              shift-right: [w412] -> w402
              shift-left: w405 -> [w414]
              n229 = local read "next-state-cluster-const"() -> (w406:T1)
              n230 = Bundle By Name(cluster=w406, "next-state"="move", "bypass-confirm"=TRUE, "PDX"=w419, "PDY"=w418, "BarX"=93.0, "BarY"=20.0, "BMA"=45.0, "PDA"=181.0) -> (w413:T1)
              n231 = Bundle By Name(cluster=w406, "next-state"="log-pd3") -> (w407:T1)
              n232 = Build Array (concatenate)(w414, w413, w407) -> (w412:T4)
            }
            n233 = Array Size(array=w402) -> (size(s)=w399:i32)
            n234 = local write "queue-size"(w399) -> ()
          }
          frame "scan-v2" {
            n235 = local read "next-state-cluster-const"() -> (w431:T1)
            n236 = call "build-scan-pts-list.vi"("Y in"="PD Y - out", "X in"="PD X - out") -> ("Y out"=w426:dbl[], "X out"=w440:dbl[])  [unwired: 8 in]
            n237 = Initialize Array(w431, 0 ("dimension size")) -> (w433:T4)
            n238 = for {
              tunnel: w440 -> [w483] mode=indexing
              tunnel: w426 -> [w482] mode=indexing
              shift-right: [w477] -> w429
              shift-left: w433 -> [w479]
              tunnel: ["out-bar-x"] -> w421 mode=indexing
              tunnel: ["out-bar-y"] -> w420 mode=indexing
              # "Bar Out PD Scan"
              n239 = local read "next-state-cluster-const"() -> (w473:T1)
              n240 = Bundle By Name(cluster=w473, "next-state"="move", "bypass-confirm"=TRUE, "PDX"=w483, "PDY"=w482, "BarX"="out-bar-x", "BarY"="out-bar-y", "BMA"="out-bma", "PDA"="out-pda", "bar-note"=FALSE) -> (w478:T1)
              n241 = Bundle By Name(cluster=w473, "next-state"="log-pd3", "bar-note"=FALSE) -> (w471:T1)
              n242 = Build Array (concatenate)(w479, w478, w471) -> (w477:T4)
            }
            n243 = disable-structure shown="Disabled" {
              frame Disabled {
                n244 = call "build-scan-pts-list.vi"("Y in"="Bar Y - in", "X in"="Bar X - in") -> ()  [unwired: 8 in, 2 out]
              }
              frame Enabled {
              }
            }
            n245 = local read "state-queue"() -> (w430:T4)
            n246 = call "build-scan-pts-list.vi"("Y in"="PD Y - in", "X in"="PD X - in") -> ("Y out"=w424:dbl[], "X out"=w425:dbl[])  [unwired: 8 in]
            n247 = for {
              tunnel: w421 -> [w451] mode=indexing
              tunnel: w420 -> [w450] mode=indexing
              shift-right: [w449] -> w427
              shift-left: w430 -> [w446]
              tunnel: w429 -> [w444]
              tunnel: w425 -> [w448]
              tunnel: w424 -> [w447]
              n248 = Build Array (concatenate)(w446, w444) -> (w445:T4)
              n249 = for {
                shift-right: [w463] -> w449
                shift-left: w445 -> [w465]
                tunnel: w451 -> [w462]
                tunnel: w450 -> [w461]
                tunnel: w448 -> [w457] mode=indexing
                tunnel: w447 -> [w456] mode=indexing
                # "Bar in PD Scan"
                n250 = local read "next-state-cluster-const"() -> (w458:T1)
                n251 = Bundle By Name(cluster=w458, "next-state"="move", "bypass-confirm"=TRUE, "PDX"=w457, "PDY"=w456, "BarX"=w462, "BarY"=w461, "BMA"="in-bma", "PDA"="in-pda", "bar-note"=TRUE) -> (w464:T1)
                n252 = Bundle By Name(cluster=w458, "next-state"="log-pd3", "bar-note"=TRUE) -> (w454:T1)
                n253 = Build Array (concatenate)(w465, w464, w454) -> (w463:T4)
              }
            }
            n254 = local read "next-state-cluster-const"() -> (w434:T1)
            n255 = Bundle By Name(cluster=w434, "next-state"="wait", "PDX"="Test Start Delay (s)") -> (w441:T1)
            n256 = Build Array (concatenate)(w441, w427) -> (w428:T4)
            n257 = Array Size(array=w428) -> (size(s)=w435:i32)
            n258 = local write "queue-size"(w435) -> ()
          }
          frame "wait" {
            n259 = property on="start-msg" class="Str"("Visible"=TRUE) -> ()  [unwired: 2 in, 2 out]
            n260 = local write "start-msg"("\n\n\nProgram Delay Active\nfor User to Exit Laser Area" ("String")) -> ()
            n261 = Unbundle By Name(w487) -> ("PDX"=w488:dbl)
            n262 = Multiply(x=w488, y=1000.0) -> (x*y=w490:dbl)
            n263 = Wait (ms)(milliseconds to wait=w490) -> ()  [unwired: 1 out]
            n264 = local read "state-queue"() -> (w486:T4)
          }
          frame "align-setup" {
            n265 = Unbundle By Name(w497) -> ("bypass-confirm"=w493:bool)
            n266 = Select(t="gr-asc", s=w493, f="nelder-mead") -> (s? t:f=w496:string)
            n267 = case shown="False" "align-only" {
              tunnel: w496 -> [w503 w509]
              tunnel: [w498 w512] -> w492
              frame False {
                n268 = local read "Test Start Delay (s)"() -> (w505:dbl)
                n269 = local read "next-state-cluster-const"() -> (w499:T1)
                n270 = local read "state-queue"() -> (w507:T4)
                n271 = Bundle By Name(cluster=w499, "next-state"="wait", "PDX"=w505) -> (w504:T1)
                n272 = Bundle By Name(cluster=w499, "next-state"=w503) -> (w501:T1)
                n273 = Bundle By Name(cluster=w499, "next-state"="diode-scan-center") -> (w500:T1)
                n274 = Build Array (concatenate)(w507, w504, w501, w500) -> (w498:T4)
              }
              frame True {
                n275 = local read "next-state-cluster-const"() -> (w508:T1)
                n276 = Bundle By Name(cluster=w508, "next-state"=w509) -> (w510:T1)
                n277 = local read "state-queue"() -> (w511:T4)
                n278 = Build Array (concatenate)(w511, w510) -> (w512:T4)
              }
            }
          }
          frame "nelder-mead" {
            n279 = property on="start-msg" class="Str"("Visible"=TRUE) -> ()  [unwired: 2 in, 2 out]
            n280 = local read "stage-error"() -> (w528:errorcluster)
            n281 = call "get-stage-positions.vi"("error in (no error)"=w528, "Cluster"=w526) -> ("error out"=w527:errorcluster, "stage positions"=w525:T2)  [unwired: 8 in]
            n282 = Unbundle By Name(w527) -> ("status"=w529:bool)
            n283 = local write "stage-error"(w527) -> ()
            n284 = local write "stage-stat"(w529) -> ()
            n285 = local read "meter-error"() -> (w533:errorcluster)
            n286 = local read "stage-error"() -> (w532:errorcluster)
            n287 = local read "meter-visa"() -> (w531:refnum<visa-resource-name>)
            n288 = local read "PD Values"() -> (w530:cluster{"PD1":dbl, "PD2":dbl, "PD3":dbl})
            n289 = local write "start-msg"("\n\n\n\nPerforming Automated\nAlignment.\n\nPlease Wait.\n" ("String")) -> ()
            n290 = Unbundle By Name(w525) -> ("PD Y"=w523:dbl, "PD X"=w524:dbl)
            n291 = Bundle By Name(cluster=T7 {"alpha"=1.0, "gamma"=2.0, "rho"=0.5, "sigma"=0.5, "simplex L"=0.5} ("NM-params"), "simplex L"=0.5, "sigma"=0.5) -> (w515:T7)
            n292 = call "auto_alignment.vi"("meter-visa"=w531, "xStart"=w524, "yStart"=w523, "NM-params"=w515, "PD Values"=w530, "stage-refs"=w526, "meter-error-in"=w533, "stage-error-in"=w532) -> ("Optimized Location"=→"Optimized Location":dbl[], "meter-error-out"=w522:errorcluster, "run time (min)"=→"run time (min)":dbl, "stage-error-out"=w521:errorcluster)  [unwired: 3 in, 1 out]
            n293 = local write "meter-error"(w522) -> ()
            n294 = local write "stage-error"(w521) -> ()
            n295 = local read "state-queue"() -> (w534:T4)
          }
          frame "multi-trial" {
            n296 = local read "next-state-cluster-const"() -> (w535:T1)
            n297 = Initialize Array(w535, 0 ("dimension size")) -> (w543:T4)
            n298 = for {
              N: 20 -> [_]
              shift-right: [w564] -> w538
              shift-left: w543 -> [w565]
              tunnel: "PDX start" -> [w551]
              tunnel: "PDY start" -> [w547]
              w546 = 2.0
              n299 = Subtract(x=w547, y=w546) -> (x-y=w548:dbl)
              n300 = Add(x=w547, y=w546) -> (x+y=w549:dbl)
              n301 = Subtract(x=w551, y=w546) -> (x-y=w553:dbl)
              n302 = Add(x=w551, y=w546) -> (x+y=w552:dbl)
              n303 = call-poly <vilib>:"Random Number (Range).vi"("lower bound (0)"=w548, "upper bound (100)"=w549) -> ("number"=w545:dbl)  [unwired: 9 in]
              n304 = call-poly <vilib>:"Random Number (Range).vi"("lower bound (0)"=w553, "upper bound (100)"=w552) -> ("number"=w550:dbl)  [unwired: 9 in]
              n305 = local read "next-state-cluster-const"() -> (w561:T1)
              n306 = Bundle By Name(cluster=w561, "next-state"="move", "bypass-confirm"=TRUE, "PDX"=w550, "PDY"=w545, "BarX"=90.0, "BarY"=35.0, "BMA"=45.0, "PDA"=181.0, "bar-note"=FALSE) -> (w562:T1)
              n307 = Bundle By Name(cluster=w561, "next-state"="nelder-mead") -> (w563:T1)
              n308 = Build Array (concatenate)(w565, w562, w563) -> (w564:T4)
            }
            n309 = Bundle By Name(cluster=w535, "next-state"="diode-scan-center") -> (w536:T1)
            n310 = Build Array (concatenate)(w538, w536) -> (w537:T4)
          }
        }
        n311 = Subtract(x=w105, y=w104) -> (x-y=→"loop-rate":u32)
        n312 = Get Date/Time In Seconds() -> (seconds since 1Jan1904=w100:timestamp)
        n313 = Format Date/Time String(time format string (%c)="%Y-%m-%d %H:%M:%S", seconds (now)=w100) -> (date/time string=→"Current Time:":string)  [unwired: 1 in]
      }
    }
    frame #4 {
      # "close stages"
      n314 = local read "main-stage-refs"() -> (w567:T3)
      n315 = Unbundle By Name(w567) -> ("Bar X main"=w573:refnum<k24>, "Bar Y main"=w572:refnum<k24>, "PD X main"=w571:refnum<k24>, "PD Y main"=w570:refnum<k24>, "BMA main"=w569:refnum<k24>, "PDA main"=w568:refnum<k24>)
      n316 = invoke class="BenchtopStepperControl" method="CloseDevice"(reference=w569) -> (error out=w578:errorcluster)  [unwired: 2 in, 2 out]
      n317 = invoke class="BenchtopStepperControl" method="CloseDevice"(reference=w568) -> (error out=w579:errorcluster)  [unwired: 2 in, 2 out]
      n318 = invoke class="LongTravelStageControl" method="CloseDevice"(reference=w573) -> (error out=w574:errorcluster)  [unwired: 2 in, 2 out]
      n319 = invoke class="LongTravelStageControl" method="CloseDevice"(reference=w572) -> (error out=w575:errorcluster)  [unwired: 2 in, 2 out]
      n320 = invoke class="LongTravelStageControl" method="CloseDevice"(reference=w571) -> (error out=w576:errorcluster)  [unwired: 2 in, 2 out]
      n321 = invoke class="LongTravelStageControl" method="CloseDevice"(reference=w570) -> (error out=w577:errorcluster)  [unwired: 2 in, 2 out]
      n322 = local read "stage-error"() -> (w580:errorcluster)
      n323 = Merge Errors(w580, w574, w575, w576, w577, w578, w579) -> (w581:errorcluster)
      n324 = local write "stage-error"(w581) -> ()
    }
    frame #5 {
      # "Close connection to meter"
      n325 = local read "meter-error"() -> (w583:errorcluster)
      n326 = local read "meter-visa"() -> (w582:refnum<visa-resource-name>)
      n327 = call <instrlib>:"Close.vi"("error in (no error)"=w583, "VISA resource name"=w582) -> ("error out"=w584:errorcluster)  [unwired: 9 in]
      n328 = local write "meter-error"(w584) -> ()
    }
    frame #6 {
      # "Section deletes log file if nothing is written to it\nto prevent just a ton of empty files during development"
      n329 = local read "log-error"() -> (w587:errorcluster)
      n330 = local read "keep-file"() -> (w585:bool)
      n331 = local read "log-path"() -> (w586:path)
      n332 = case shown="False" w585 {
        tunnel: w587 -> [w590 w592]
        tunnel: [w591 w592] -> w588
        tunnel: w586 -> [w589 _]
        frame False {
          n333 = Delete(path (use dialog)=w589, error in=w590) -> (error out=w591:errorcluster)  [unwired: 3 in, 2 out]
        }
        frame True {
        }
      }
      n334 = local write "log-error"(w588) -> ()
    }
  }
